vi "SSC Digital Stream HRAM Results.vi"(0 "Digital SSC in":T3[](array[typedef]), 11 "error in":errorcluster) -> (4 "Digital SSC out":T3[](array[typedef]), 6 "per-instrument per-site cycle information":T1[][](array[typedef]) {"actual pin states" items=["0"=0, "1"=1, "L"=3, "H"=4, "X"=5, "M"=6, "V"=7, "D"=8, "E"=9, "Not A Pin State"=254, "Pin State Not Acquired"=255]; "expected pin states" items=["0"=0, "1"=1, "L"=3, "H"=4, "X"=5, "M"=6, "V"=7, "D"=8, "E"=9, "Not A Pin State"=254, "Pin State Not Acquired"=255]}, 8 "per-instrument per-site scan cycle numbers":i64[][](array[numeric]), 10 "number of samples":i64, 15 "error out":errorcluster)   [LabVIEW 2019]
doc: "Measures the frequency on the specified pin(s) and pin group(s) over the configured measurement time."
uses:
  SSC Digital.ctl
  <instrlib>/niDigital/niDigital.llb/niDigital History RAM Cycle Information (1D Pin States).ctl
  <instrlib>/niDigital/niDigital.llb/niDigital Pin State.ctl
  Shared SubVIs/Site List to Site Numbers.vi
  Shared SubVIs/Channel List to Pins.vi
  Shared SubVIs/Trim Whitespace [Inlined].vi
  <instrlib>/niDigital/niDigital.llb/niDigital Fetch History RAM Cycle Information (1D Pin States).vi
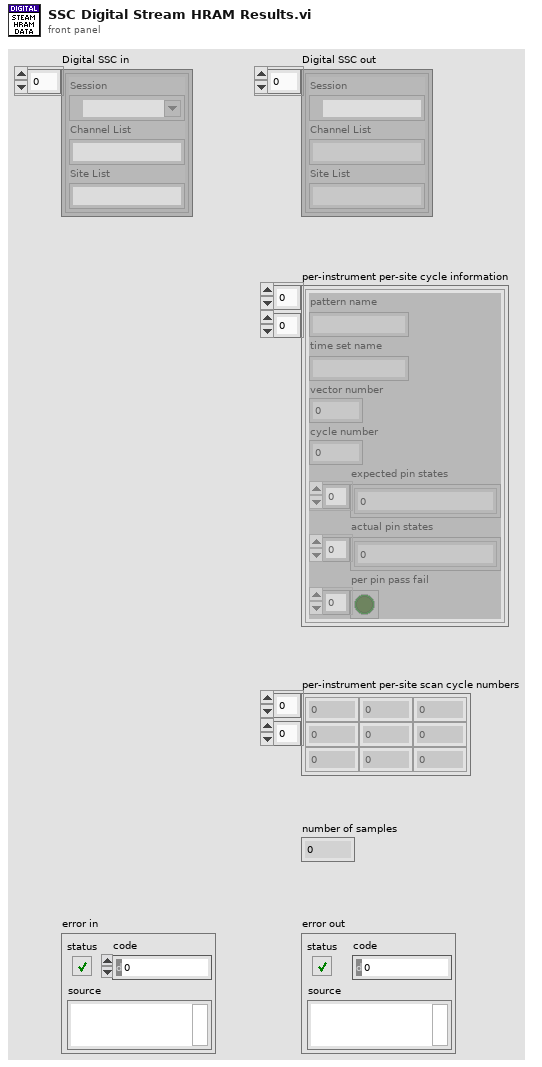
[diagram p1: front panel]
types:
  T1 = typedef "niDigital History RAM Cycle Information (1D Pin States).ctl" = cluster{"pattern name":string, "time set name":string, "vector number":i64, "cycle number":i64, "expected pin states":T2[], "actual pin states":T2[], "per pin pass fail":bool[]}
  T2 = typedef "niDigital Pin State.ctl" = u8
  T3 = typedef "SSC Digital.ctl" = cluster{"Session":refnum<k15>, "Channel List":string, "Site List":string}
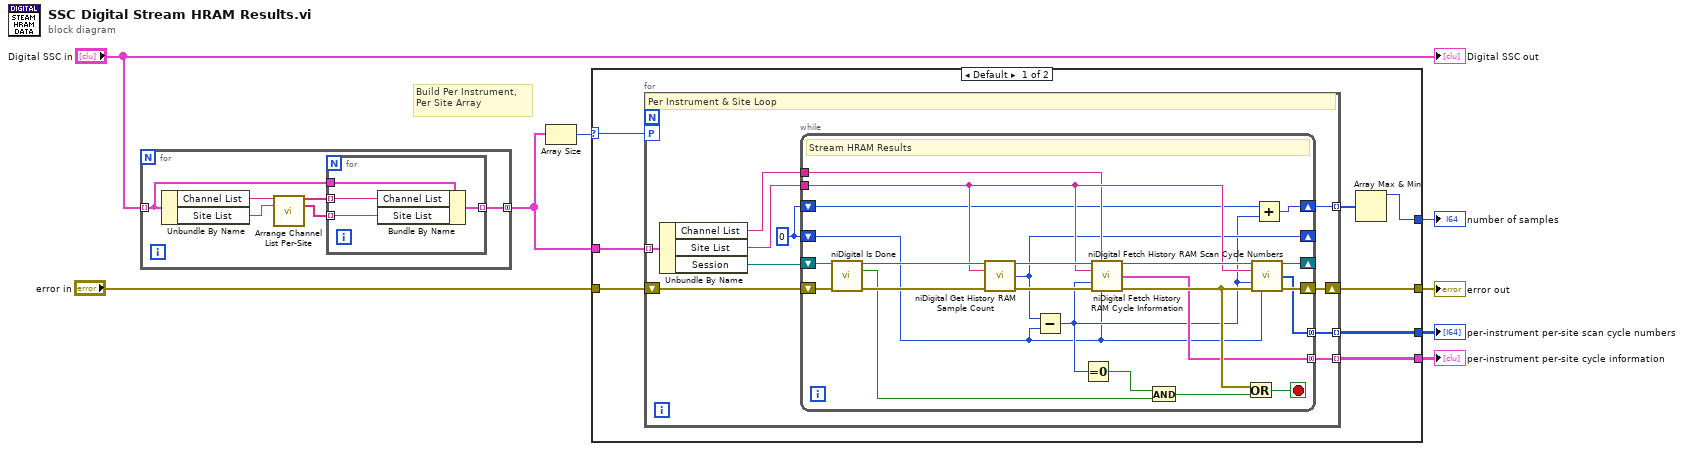
[diagram p0: block diagram]
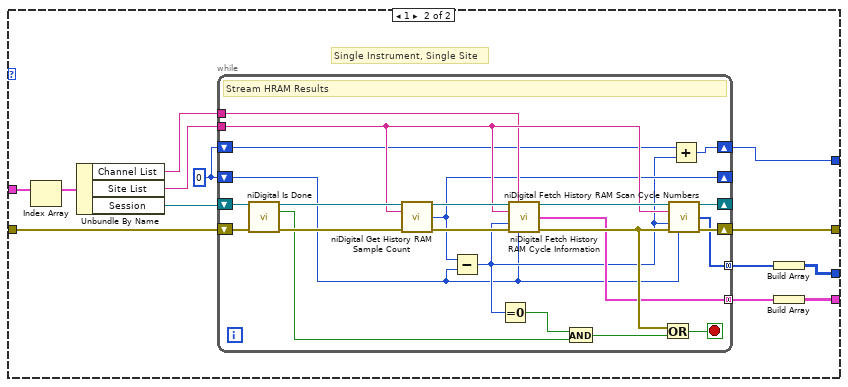
[diagram p2: hidden frame]
diagram:
  # "Build Per Instrument, Per Site Array"
  n1 = for {
    tunnel: "Digital SSC in" -> [w10] mode=indexing
    tunnel: [w9] -> w3 mode=concatenating
    n2 = Unbundle By Name(w10) -> ("Channel List"=w13:string, "Site List"=w14:string)
    n3 = call "Arrange Channel List Per-Site.vi"("Channel List String"=w13, "Site List String"=w14) -> ("Channel List Array"=w12:string[], "Site List Array"=w11:string[])  [unwired: 11 in, 1 out]
    n4 = for {
      tunnel: w12 -> [w18] mode=indexing
      tunnel: w11 -> [w17] mode=indexing
      tunnel: [w16] -> w9 mode=indexing
      tunnel: w10 -> [w15]
      n5 = Bundle By Name(cluster=w15, "Channel List"=w18, "Site List"=w17) -> (w16:T3)
    }
  }
  n6 = Array Size(array=w3) -> (size(s)=w6:i32)
  n7 = case shown="Default" w6 {
    selector: w6 -> [w23 _]
    tunnel: "error in" -> [w25 w71]
    tunnel: [w24 w70] -> w7
    tunnel: w3 -> [w26 w72]
    tunnel: [w21 w61] -> w2
    tunnel: [w22 w60] -> w1
    tunnel: [w19 w67] -> w5
    frame Default {
      n8 = for {
        tunnel: w26 -> [w36] mode=indexing
        tunnel: [w32] -> w21 mode=indexing
        tunnel: [w31] -> w22 mode=indexing
        shift-right: [w29] -> w24
        shift-left: w25 -> [w30]
        workers-P: w23 -> [_]
        tunnel: [w27] -> w20 mode=indexing
        w28 = i64 0
        # "Per Instrument & Site Loop"
        n9 = Unbundle By Name(w36) -> ("Channel List"=w33:string, "Site List"=w34:string, "Session"=w35:refnum<k15>)
        n10 = while {
          tunnel: [w49] -> w31 mode=concatenating
          tunnel: [w43] -> w32 mode=concatenating
          shift-right: [w42] -> _
          shift-left: w28 -> [w37]
          tunnel: w34 -> [w50]
          shift-right: [w48] -> _
          shift-left: w35 -> [w47]
          shift-right: [w46] -> w29
          shift-left: w30 -> [w45]
          tunnel: w33 -> [w44]
          shift-right: [w41] -> w27
          shift-left: w28 -> [w40]
          stop <- w38 stop-if-true
          # "Stream HRAM Results"
          n11 = call <instrlib>:"niDigital Is Done.vi"("instrument handle"=w47, "error in"=w45) -> ("instrument handle out"=w57:refnum<k15>, "done"=w52:bool, "error out"=w56:errorcluster)  [unwired: 11 in]
          n12 = call <instrlib>:"niDigital Get History RAM Sample Count.vi"("instrument handle"=w57, "site"=w50, "error in"=w56) -> ("instrument handle out"=w55:refnum<k15>, "sample count"=w42:i64, "error out"=w54:errorcluster)  [unwired: 10 in]
          n13 = Subtract(x=w42, y=w37) -> (x-y=w39:i64)
          n14 = Equal To 0?(x=w39) -> (x = 0?=w53:bool)
          n15 = call-poly <instrlib>:"niDigital Fetch History RAM Cycle Information.vi"("instrument handle"=w55, "pin list"=w44, "site"=w50, "samples to read (-1)"=w39, "error in"=w54, "position"=w37) -> ("instrument handle out"=w58:refnum<k15>, "cycle information"=w49:T1[], "error out"=w59:errorcluster)  [unwired: 7 in]
          n16 = And(x=w53, y=w52) -> (x .and. y?=w51:bool)
          n17 = Or(x=w59, y=w51) -> (x .or. y?=w38:bool)
          n18 = call <instrlib>:"niDigital Fetch History RAM Scan Cycle Numbers.vi"("instrument handle"=w58, "site"=w50, "samples to read (-1)"=w39, "error in"=w59, "position"=w37) -> ("instrument handle out"=w48:refnum<k15>, "scan cycle numbers"=w43:i64[], "error out"=w46:errorcluster)  [unwired: 8 in]
          n19 = Add(x=w40, y=w39) -> (x+y=w41:i64)
        }
      }
      n20 = Array Max & Min(array=w20) -> (max value=w19:i64)  [unwired: 3 out]
    }
    frame 1 {
      w63 = i64 0
      # "Single Instrument, Single Site"
      n21 = Index Array(array=w72) -> (element=w62:T3)  [unwired: 1 in]
      n22 = Unbundle By Name(w62) -> ("Channel List"=w64:string, "Site List"=w65:string, "Session"=w66:refnum<k15>)
      n23 = while {
        tunnel: [w85] -> w69 mode=concatenating
        tunnel: [w79] -> w68 mode=concatenating
        shift-right: [w78] -> _
        shift-left: w63 -> [w73]
        tunnel: w65 -> [w86]
        shift-right: [w84] -> _
        shift-left: w66 -> [w83]
        shift-right: [w82] -> w70
        shift-left: w71 -> [w81]
        tunnel: w64 -> [w80]
        shift-right: [w77] -> w67
        shift-left: w63 -> [w76]
        stop <- w74 stop-if-true
        # "Stream HRAM Results"
        n24 = call <instrlib>:"niDigital Is Done.vi"("instrument handle"=w83, "error in"=w81) -> ("instrument handle out"=w93:refnum<k15>, "done"=w88:bool, "error out"=w92:errorcluster)  [unwired: 11 in]
        n25 = call <instrlib>:"niDigital Get History RAM Sample Count.vi"("instrument handle"=w93, "site"=w86, "error in"=w92) -> ("instrument handle out"=w91:refnum<k15>, "sample count"=w78:i64, "error out"=w90:errorcluster)  [unwired: 10 in]
        n26 = Subtract(x=w78, y=w73) -> (x-y=w75:i64)
        n27 = Equal To 0?(x=w75) -> (x = 0?=w89:bool)
        n28 = call-poly <instrlib>:"niDigital Fetch History RAM Cycle Information.vi"("instrument handle"=w91, "pin list"=w80, "site"=w86, "samples to read (-1)"=w75, "error in"=w90, "position"=w73) -> ("instrument handle out"=w94:refnum<k15>, "cycle information"=w85:T1[], "error out"=w95:errorcluster)  [unwired: 7 in]
        n29 = And(x=w89, y=w88) -> (x .and. y?=w87:bool)
        n30 = Or(x=w95, y=w87) -> (x .or. y?=w74:bool)
        n31 = call <instrlib>:"niDigital Fetch History RAM Scan Cycle Numbers.vi"("instrument handle"=w94, "site"=w86, "samples to read (-1)"=w75, "error in"=w95, "position"=w73) -> ("instrument handle out"=w84:refnum<k15>, "scan cycle numbers"=w79:i64[], "error out"=w82:errorcluster)  [unwired: 8 in]
        n32 = Add(x=w76, y=w75) -> (x+y=w77:i64)
      }
      n33 = Build Array(w68) -> (w61:i64[][])
      n34 = Build Array(w69) -> (w60:T1[][])
    }
  }
  "error out" <- w7
  "per-instrument per-site scan cycle numbers" <- w2
  "per-instrument per-site cycle information" <- w1
  "number of samples" <- w5
  "Digital SSC out" <- "Digital SSC in"
